vi "Add.vi"(1 "Password":string, 2 "Username":string, 3 "Datos":string) -> (0 "Added":bool)   [LabVIEW 2017]
doc: "Verifica si el usuario está en la base de datos"
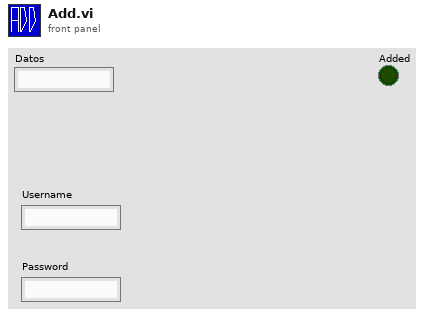
[diagram p1: front panel]
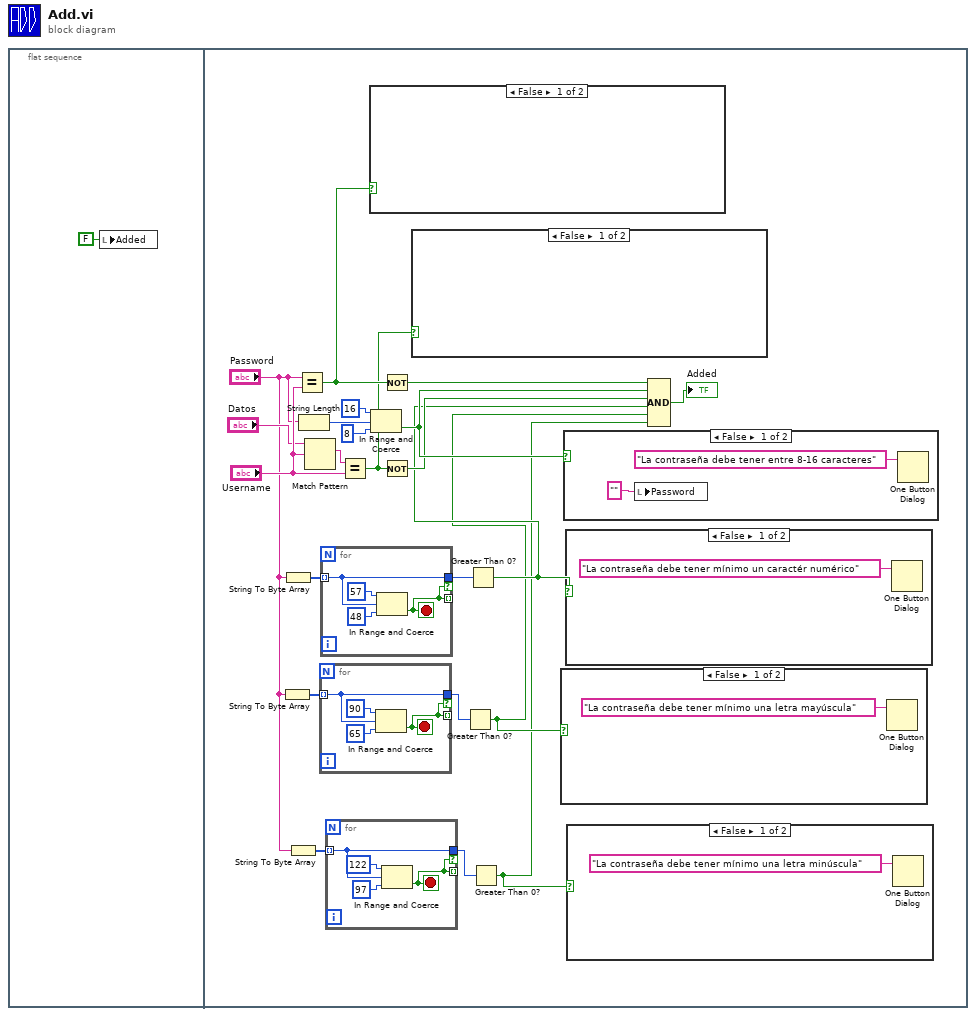
[diagram p0: block diagram]
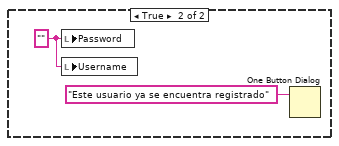
[diagram p5: hidden frame]
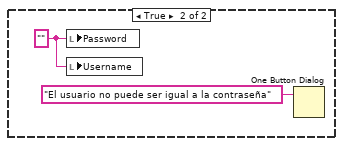
[diagram p6: hidden frame]
diagram:
  n1 = flat-sequence {
    frame #0 {
      n2 = local write "Added"(FALSE ("result")) -> ()
    }
    frame #1 {
      n3 = String To Byte Array(string="Password") -> (unsigned byte array=w8:u8[])
      n4 = String To Byte Array(string="Password") -> (unsigned byte array=w11:u8[])
      n5 = String To Byte Array(string="Password") -> (unsigned byte array=w4:u8[])
      n6 = Equal?(x="Password", y="Username") -> (x = y?=w18:bool)
      n7 = String Length(string="Password") -> (length=w23:i32)
      n8 = Match Pattern(string="Datos", regular expression="Username") -> (match substring=w17:string)  [unwired: 1 in, 3 out]
      n9 = for {
        tunnel: w8 -> [w30] mode=indexing
        tunnel: [w30] -> w7 if=w31
        tunnel: [w31] -> _ mode=indexing
        stop <- w31 stop-if-true
        n10 = In Range and Coerce(upper limit=u8 90, x=w30, lower limit=u8 65) -> (In Range?=w31:bool)  [unwired: 1 out]
      }
      n11 = for {
        tunnel: w11 -> [w35] mode=indexing
        tunnel: [w35] -> w10 if=w36
        tunnel: [w36] -> _ mode=indexing
        stop <- w36 stop-if-true
        n12 = In Range and Coerce(upper limit=u8 57, x=w35, lower limit=u8 48) -> (In Range?=w36:bool)  [unwired: 1 out]
      }
      n13 = for {
        tunnel: w4 -> [w25] mode=indexing
        tunnel: [w25] -> w5 if=w26
        tunnel: [w26] -> _ mode=indexing
        stop <- w26 stop-if-true
        n14 = In Range and Coerce(upper limit=u8 122, x=w25, lower limit=u8 97) -> (In Range?=w26:bool)  [unwired: 1 out]
      }
      n15 = Equal?(x=w17, y="Username") -> (x = y?=w15:bool)
      n16 = case shown="False" w18 {
        frame False {
        }
        frame True {
          w41 = "" ("Username")
          n17 = local write "Password"(w41) -> ()
          n18 = local write "Username"(w41) -> ()
          n19 = One Button Dialog(message="El usuario no puede ser igual a la contraseña") -> ()  [unwired: 1 in, 1 out]
        }
      }
      n20 = In Range and Coerce(upper limit=16, x=w23, lower limit=8) -> (In Range?=w19:bool)  [unwired: 1 out]
      n21 = Not(x=w18) -> (.not. x?=w20:bool)
      n22 = Not(x=w15) -> (.not. x?=w16:bool)
      n23 = case shown="False" w15 {
        frame False {
        }
        frame True {
          w39 = "" ("Username")
          n24 = local write "Password"(w39) -> ()
          n25 = local write "Username"(w39) -> ()
          n26 = One Button Dialog(message="Este usuario ya se encuentra registrado") -> ()  [unwired: 1 in, 1 out]
        }
      }
      n27 = Greater Than 0?(x=w7) -> (x > 0?=w6:bool)
      n28 = Greater Than 0?(x=w10) -> (x > 0?=w9:bool)
      n29 = Greater Than 0?(x=w5) -> (x > 0?=w2:bool)
      n30 = case shown="False" w6 {
        frame False {
          n31 = One Button Dialog(message="La contraseña debe tener mínimo una letra mayúscula") -> ()  [unwired: 1 in, 1 out]
        }
        frame True {
        }
      }
      n32 = case shown="False" w19 {
        frame False {
          n33 = local write "Password"("" ("Username")) -> ()
          n34 = One Button Dialog(message="La contraseña debe tener entre 8-16 caracteres") -> ()  [unwired: 1 in, 1 out]
        }
        frame True {
        }
      }
      n35 = case shown="False" w9 {
        frame False {
          n36 = One Button Dialog(message="La contraseña debe tener mínimo un caractér numérico") -> ()  [unwired: 1 in, 1 out]
        }
        frame True {
        }
      }
      n37 = case shown="False" w2 {
        frame False {
          n38 = One Button Dialog(message="La contraseña debe tener mínimo una letra minúscula") -> ()  [unwired: 1 in, 1 out]
        }
        frame True {
        }
      }
      n39 = Compound Arithmetic op=AND(w20, w19, w16, w9, w6, w2) -> (→"Added":bool)
    }
  }
